vi "Measure Output.vi"(8 "error in":errorcluster, 11 "Acopian in":refnum<class "Acopian.lvclass">) -> (0 "error out":errorcluster, 1 "Current":dbl[](array[numeric]), 2 "Voltage":dbl[](array[numeric]), 3 "Acopian out":refnum<class "Acopian.lvclass">)   [LabVIEW 2019, in "Acopian.lvlib" / "Acopian.lvclass"]
doc: "Child classes must override this VI:\n\nThis VI is the device specific query of current and voltage measurements. \nThe return values are: \nVoltage Array - One voltage measurement per channel single channel supplies should only return a single array element\nCurrent Array - - One current measurement per channel single channel supplies should only return a single array element"
uses:
  Library/Acopian.lvclass
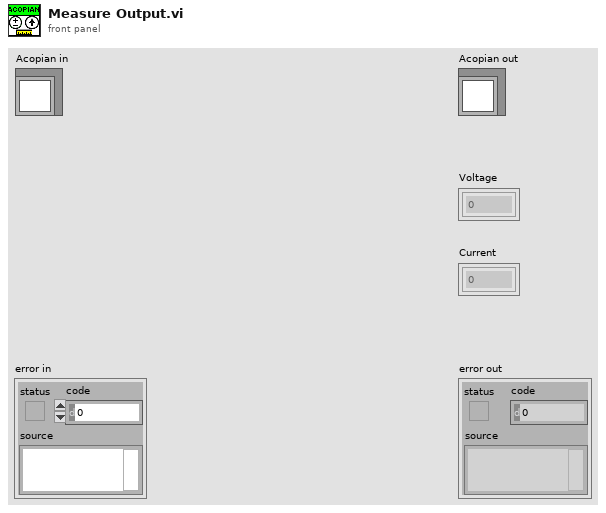
[diagram p1: front panel]
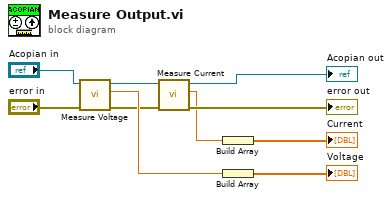
[diagram p0: block diagram]
diagram:
  n1 = call "Measure Voltage.vi"("error in"="error in", "Acopian in"="Acopian in") -> ("error out"=w5:errorcluster, "Voltage"=w8:dbl, "Acopian out"=w6:refnum<class "Acopian.lvclass">)  [unwired: 7 in]
  n2 = call "Measure Current.vi"("error in"=w5, "Acopian in"=w6) -> ("error out"=→"error out":errorcluster, "Current"=w2:dbl, "Acopian out"=→"Acopian out":refnum<class "Acopian.lvclass">)  [unwired: 7 in]
  n3 = Build Array(w2) -> (→"Current":dbl[])
  n4 = Build Array(w8) -> (→"Voltage":dbl[])
